vi "ex5-4.vi"   [LabVIEW 2014]
uses:
  <vilib>/NXT/Dual Mode Library/Motors/MotorOn.vi
  <vilib>/NXT/Dual Mode Library/Waits/Wait_Rotation.vi
  <vilib>/NXT/Dual Mode Library/Motors/MotorBrake.vi
types:
  T1 = typedef "LVHSConnector.ctl" = refnum<class "BrickReference.lvclass">
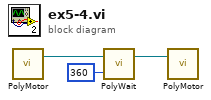
[diagram p0: block diagram]
diagram:
  n1 = call-poly <vilib>:"PolyMotor.vi"() -> ("NXT/EV3"=w3:T1)  [unwired: 4 in]
  n2 = call-poly <vilib>:"PolyWait.vi"("Position Change (180)"=360, "NXT/EV3"=w3) -> ("NXT/EV3"=w2:T1)  [unwired: 2 in]
  n3 = call-poly <vilib>:"PolyMotor.vi"("NXT/EV3"=w2) -> ()  [unwired: 3 in, 1 out]
